vi "Joystick Driver Controls OLD.vi"(4 "Shift Value":T1, 7 "X":dbl, 10 "Throttle":dbl, 11 "Y":dbl) -> (2 "Y":dbl, 3 "X":dbl)   [LabVIEW 2017]
uses:
  <vilib>/Rock Robotics/WPI/Solenoid/WPI_SolenoidValue.ctl
  <vilib>/Rock Robotics/Network Tables/NT Read Number.vi
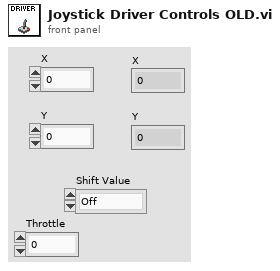
[diagram p1: front panel]
types:
  T1 = typedef "WPI_SolenoidValue.ctl" = enum16{"Off", "On", "Forward", "Reverse"}
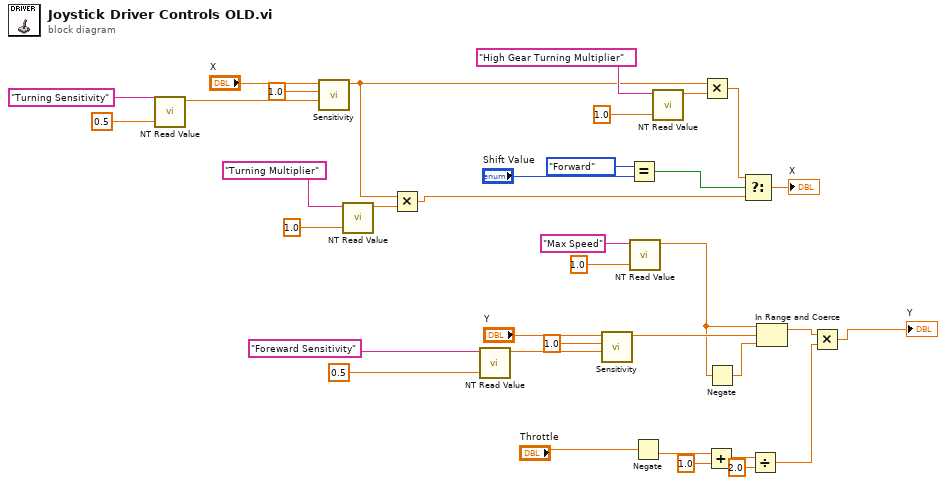
[diagram p0: block diagram]
diagram:
  n1 = call-poly <vilib>:"NT Read Value.vi"("Default Value"=0.5, "Name"="Turning Sensitivity") -> ("Numeric"=w20:dbl)  [unwired: 8 in, 1 out]
  n2 = call "Sensitivity.vi"("Power (z)"=w20, "Sensitivity (a)"=1.0, "Input"="X") -> ("Output"=w10:dbl)  [unwired: 8 in]
  n3 = call-poly <vilib>:"NT Read Value.vi"("Default Value"=1.0, "Name"="Turning Multiplier") -> ("Numeric"=w11:dbl)  [unwired: 8 in, 1 out]
  n4 = Multiply(x=w10, y=w11) -> (x*y=w9:dbl)
  n5 = call-poly <vilib>:"NT Read Value.vi"("Default Value"=0.5, "Name"="Foreward Sensitivity") -> ("Numeric"=w18:dbl)  [unwired: 8 in, 1 out]
  n6 = call "Sensitivity.vi"("Power (z)"=w18, "Sensitivity (a)"=1.0, "Input"="Y") -> ("Output"=w35:dbl)  [unwired: 8 in]
  n7 = Equal?(x=WPI_SolenoidValue."Forward", y="Shift Value") -> (x = y?=w28:bool)
  n8 = call-poly <vilib>:"NT Read Value.vi"("Default Value"=1.0, "Name"="Max Speed") -> ("Numeric"=w14:dbl)  [unwired: 8 in, 1 out]
  n9 = Negate(x="Throttle") -> (-x=w8:dbl)
  n10 = call-poly <vilib>:"NT Read Value.vi"("Default Value"=1.0, "Name"="High Gear Turning Multiplier") -> ("Numeric"=w23:dbl)  [unwired: 8 in, 1 out]
  n11 = Multiply(x=w10, y=w23) -> (x*y=w29:dbl)
  n12 = Add(x=w8, y=1.0) -> (x+y=w6:dbl)
  n13 = Negate(x=w14) -> (-x=w36:dbl)
  n14 = Select(t=w29, s=w28, f=w9) -> (s? t:f=→"X":dbl)
  n15 = Divide(x=w6, y=2.0) -> (x/y=w2:dbl)
  n16 = In Range and Coerce(upper limit=w14, x=w35, lower limit=w36) -> (coerced(x)=w3:dbl)  [unwired: 1 out]
  n17 = Multiply(x=w3, y=w2) -> (x*y=→"Y":dbl)
